vi "Serial Write.vi"(8 "error in":errorcluster, 9 "timeout (ms)":i32, 10 "data":u8[](array[numeric]), 11 "Visa Resource":refnum<visa-resource-name>) -> (0 "error out":errorcluster, 1 "timed out?":bool)   [LabVIEW 2021, in "Serial Shared Components.lvlib"]
doc: "Performs a write on the serial port."
uses:
  Serial Shared Components.lvlib
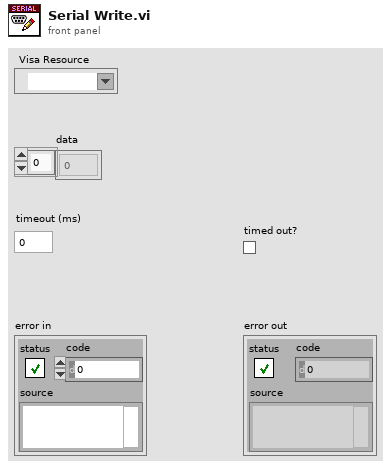
[diagram p1: front panel]
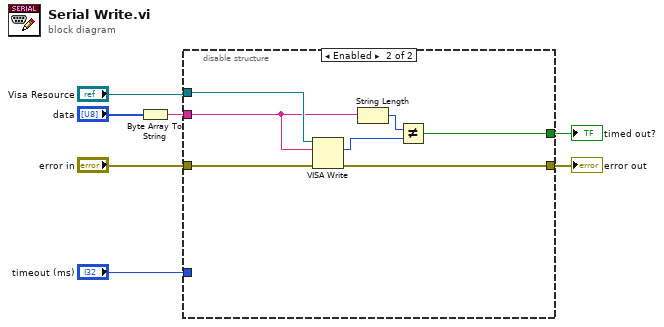
[diagram p0: block diagram]
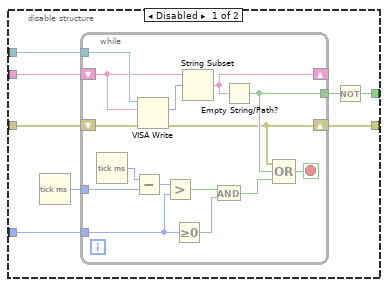
[diagram p2: hidden frame]
diagram:
  n1 = Byte Array To String(unsigned byte array="data") -> (string=w3:string)
  n2 = disable-structure shown="Enabled" {
    disable-tunnel: "timeout (ms)" -> [w15 _]
    disable-tunnel: "error in" -> [w14 w37]
    disable-tunnel: [w13 w36] -> w5
    disable-tunnel: "Visa Resource" -> [w12 w35]
    disable-tunnel: [w11 w31] -> w6
    disable-tunnel: w3 -> [w9 w34]
    frame Disabled {
      n3 = Tick Count (ms)() -> (millisecond timer value=w8:u32)
      n4 = while {
        tunnel: w8 -> [w28]
        shift-right: [w16] -> w13
        shift-left: w14 -> [w22]
        tunnel: [w18] -> w10
        tunnel: w15 -> [w24]
        tunnel: w12 -> [w21]
        shift-right: [w17] -> _
        shift-left: w9 -> [w20]
        stop <- w30 stop-if-true
        n5 = Tick Count (ms)() -> (millisecond timer value=w29:u32)
        n6 = Subtract(x=w29, y=w28) -> (x-y=w26:u32)
        n7 = VISA Write(VISA resource name=w21, write buffer=w20, error in (no error)=w22) -> (return count=w19:u32, error out=w16:errorcluster)  [unwired: 1 out]
        n8 = Greater?(x=w26, y=w24) -> (0:w25:bool)
        n9 = Greater Or Equal To 0?(x=w24) -> (x >= 0?=w23:bool)
        n10 = String Subset(string=w20, offset (0)=w19) -> (substring=w17:string)  [unwired: 1 in]
        n11 = And(x=w25, y=w23) -> (x .and. y?=w27:bool)
        n12 = Empty String/Path?(string/path=w17) -> (empty?=w18:bool)
        n13 = Compound Arithmetic op=OR(w16, w18, w27) -> (w30:bool)
      }
      n14 = Not(x=w10) -> (.not. x?=w11:bool)
    }
    frame Enabled {
      n15 = VISA Write(VISA resource name=w35, write buffer=w34, error in (no error)=w37) -> (return count=w33:u32, error out=w36:errorcluster)  [unwired: 1 out]
      n16 = String Length(string=w34) -> (length=w32:i32)
      n17 = Not Equal?(x=w32, y=w33) -> (x != y?=w31:bool)
    }
  }
  "timed out?" <- w6
  "error out" <- w5
